vi "tearDown.vi"(8 "error in (no error)":errorcluster, 11 "reference in":refnum<class "TestCSMSuite.lvclass">) -> (0 "error out":errorcluster, 3 "reference out":refnum<class "TestCSMSuite.lvclass">)   [LabVIEW 2017, in "TestCSMSuite.lvclass"]
doc: "tearDown runs after the test method has completed. Use this method to clean up any operations or references that were opened by setUp or the test method. Unit tests should be independent of other unit tests so this VI should ensure that the next test can run in a 'clean' test environment."
uses:
  TestCSMSuite.lvclass
  src/user.lib/_NEVSTOP/Communicable State Machine(CSM)/_Support/Typedef/_CSM_List Module Scope.ctl
  TestCSMSuite.lvclass/TestCSMSuite.ctl
  src/user.lib/_NEVSTOP/Communicable State Machine(CSM)/_Support/GlobalEvent/LogFilter/LogFilter.lvclass/LogFilter.ctl
  src/user.lib/_NEVSTOP/Communicable State Machine(CSM)/AdvanceAPI/CSM - Convert Error to Argument.vi
  src/user.lib/_NEVSTOP/Communicable State Machine(CSM)/_Support/GlobalEvent/GEvt-Generate with Rule Check.vi
  src/user.lib/_NEVSTOP/Communicable State Machine(CSM)/_Support/GlobalEvent/Cache-GEvt Filter Object.vi
  src/user.lib/_NEVSTOP/Communicable State Machine(CSM)/_Support/GlobalEvent/Cache-GEvt Refs.vi
  src/user.lib/_NEVSTOP/Communicable State Machine(CSM)/AdvanceAPI/CSM - Make String Arguments Safe.vi
  src/user.lib/_NEVSTOP/Communicable State Machine(CSM)/_Support/GlobalEvent/GEvt-Convert Filter Rules - v1.2.vi
  src/user.lib/_NEVSTOP/Communicable State Machine(CSM)/_Support/ChangeFlag/FlagInstance-GEvt Filter.vi
  src/user.lib/_NEVSTOP/Communicable State Machine(CSM)/_Support/ChangeFlag/FlagInstance-GEvt Refs.vi
  src/user.lib/_NEVSTOP/Communicable State Machine(CSM)/AdvanceAPI/CSM - Keywords.vi
  src/user.lib/_NEVSTOP/Communicable State Machine(CSM)/_Support/GlobalEvent/LogFilter/SettingVIs/Set Global CSM Filter.vi
  src/user.lib/_NEVSTOP/Communicable State Machine(CSM)/_Support/GlobalEvent/LogFilter/SettingVIs/Set Global LogType Filter.vi
  src/user.lib/_NEVSTOP/Communicable State Machine(CSM)/_Support/GlobalEvent/LogFilter/SettingVIs/Set Global State Filter.vi
  src/user.lib/_NEVSTOP/Communicable State Machine(CSM)/_Support/GlobalEvent/LogFilter/SettingVIs/Set CSM LogType Filter.vi
  src/user.lib/_NEVSTOP/Communicable State Machine(CSM)/_Support/GlobalEvent/LogFilter/SettingVIs/Set CSM State Filter.vi
  src/user.lib/_NEVSTOP/Communicable State Machine(CSM)/_Support/GlobalEvent/LogFilter/SettingVIs/Set Global StateType Filter.vi
  src/user.lib/_NEVSTOP/Communicable State Machine(CSM)/_Support/GlobalEvent/LogFilter/SettingVIs/Set CSM StateType Filter.vi
  src/user.lib/_NEVSTOP/Communicable State Machine(CSM)/_Support/GlobalEvent/LogFilter/SettingVIs/Set Periodic Log Filter.vi
  src/user.lib/_NEVSTOP/Communicable State Machine(CSM)/_Support/GlobalEvent/LogFilter/SettingVIs/Set CSM Broadcast Filter.vi
  src/user.lib/_NEVSTOP/Communicable State Machine(CSM)/_Support/GlobalEvent/LogFilter/SettingVIs/Set Global Broadcast Filter.vi
  src/user.lib/_NEVSTOP/Communicable State Machine(CSM)/_Support/GlobalEvent/LogFilter/SettingVIs/Set Global UserLog Filter.vi
  src/user.lib/_NEVSTOP/Communicable State Machine(CSM)/_Support/GlobalEvent/LogFilter/SettingVIs/Set CSM UserLog Filter.vi
  src/user.lib/_NEVSTOP/Communicable State Machine(CSM)/_Support/ChangeFlag/ChangeFlag-Read.vi
  src/user.lib/_NEVSTOP/Communicable State Machine(CSM)/_Support/ChangeFlag/ChangeFlagDB.vi
  src/user.lib/_NEVSTOP/Communicable State Machine(CSM)/_Support/GlobalEvent/FGV-GlobalEventRef(lvlibp).vi
  src/user.lib/_NEVSTOP/Communicable State Machine(CSM)/_Support/GlobalEvent/FGV-GlobalEventQueues(lvlibp).vi
  src/user.lib/_NEVSTOP/Communicable State Machine(CSM)/_Support/GlobalEvent/GEvt-Valid Subscribers.vi
  src/user.lib/_NEVSTOP/Communicable State Machine(CSM)/_Support/GlobalEvent/FGV-GEvt Filter Rules(lvlibp).vi
  src/user.lib/_NEVSTOP/Communicable State Machine(CSM)/_Support/GlobalEvent/LogFilter/LogFilter - Check.vi
  src/user.lib/_NEVSTOP/Communicable State Machine(CSM)/_Support/GlobalEvent/LogFilter/LogFilter.lvclass
  src/user.lib/_NEVSTOP/Communicable State Machine(CSM)/Communicable State Machine.lvlib
panel:
  out "CSM names":string[](array[string])
  out "Module Names":string[](array[string])
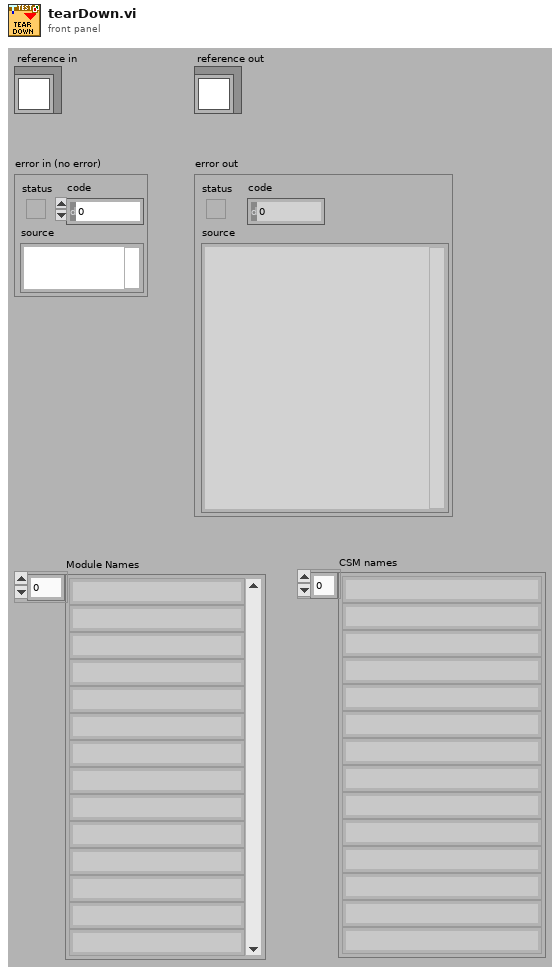
[diagram p1: front panel]
types:
  T1 = typedef "Communicable State Machine.lvlib/_CSM_List Module Scope.ctl" = enum16{"Normal", "System Only", "All"}
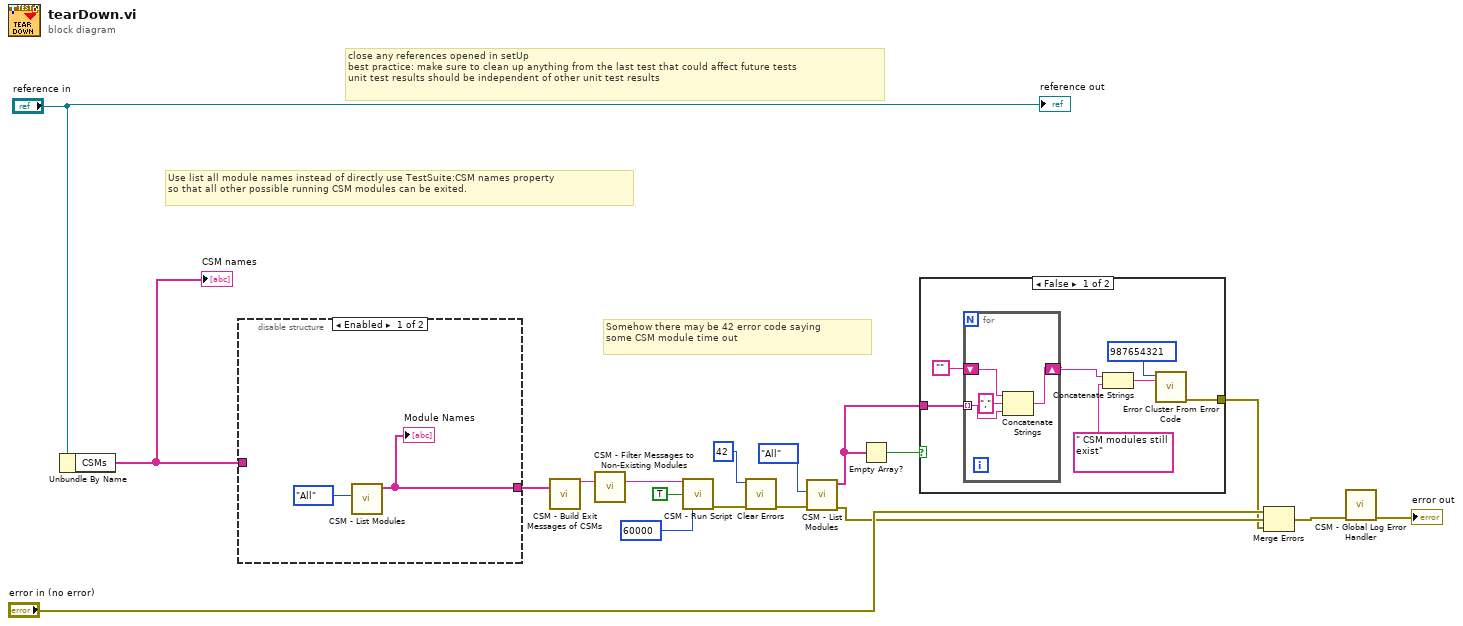
[diagram p0: block diagram]
diagram:
  # "Somehow there may be 42 error code saying\nsome CSM module time out"
  # "Use list all module names instead of directly use TestSuite:CSM names property\nso that all other possible running CSM modules can be exited."
  # "close any references opened in setUp\nbest practice: make sure to clean up anything from the last test that could affect future tests\nunit test results should be independent of other unit test results"
  n1 = Unbundle By Name("reference in") -> ("CSMs"=w12:string[])
  "CSM names" <- w12
  n2 = disable-structure shown="Enabled" {
    disable-tunnel: [w20 w21] -> w13
    disable-tunnel: w12 -> [_ w21]
    frame Enabled {
      n3 = call "CSM - List Modules.vi"("Scope (Normal)"=_CSM_List_Module_Scope."All") -> ("Module Names"=w20:string[])  [unwired: 9 in, 1 out]
      "Module Names" <- w20
    }
    frame Disabled {
    }
  }
  n4 = call "CSM - Build Exit Messages of CSMs.vi"("CSMs"=w13) -> ("States"=w16:string)  [unwired: 14 in]
  n5 = call "CSM - Filter Messages to Non-Existing Modules.vi"("States In"=w16) -> ("States Out"=w14:string)  [unwired: 14 in]
  n6 = call "CSM - Run Script.vi"("CSM Scripts"=w14, "Continue If Error? (F)"=TRUE, "Response Timeout (-2 Using Global Settings)"=60000) -> ("error out"=w10:errorcluster)  [unwired: 10 in, 2 out]
  n7 = call <vilib>:"Clear Errors.vi"("error in (no error)"=w10, "specific error code to clear (0: all)"=42) -> ("error out"=w7:errorcluster)  [unwired: 4 in, 1 out]
  n8 = call "CSM - List Modules.vi"("Error In"=w7, "Scope (Normal)"=_CSM_List_Module_Scope."All") -> ("error out"=w6:errorcluster, "Module Names"=w4:string[])  [unwired: 8 in]
  n9 = Empty Array?(array=w4) -> (empty?=w5:bool)
  n10 = case shown="False" w5 {
    tunnel: w4 -> [w28 _]
    tunnel: [w25 _] -> w3
    frame False {
      n11 = for {
        tunnel: w28 -> [w31] mode=indexing
        shift-right: [w30] -> w23
        shift-left: "" -> [w29]
        n12 = Concatenate Strings(w29, "," ("string"), w31) -> (w30:string)
      }
      n13 = Concatenate Strings(w23, " CSM modules still exist" ("string")) -> (w24:string)
      n14 = call <vilib>:"Error Cluster From Error Code.vi"("error message (\"\")"=w24, "error code (0)"=987654321) -> ("error out"=w25:errorcluster)  [unwired: 7 in]
    }
    frame True {
    }
  }
  n15 = Merge Errors("error in (no error)", w6, w3) -> (w18:errorcluster)
  n16 = call "CSM - Global Log Error Handler.vi"("Error In"=w18) -> ("error out"=→"error out":errorcluster)  [unwired: 10 in]
  "reference out" <- "reference in"
